vi "Olcme_Enstrumantasyon_Proje_170519035.vi"() -> ()   [LabVIEW 2021]
uses:
  <vilib>/Instr/_visa.llb/VISA Configure Serial Port (Instr).vi
panel:
  out "Z Ekseni İvme":dbl
  out "Y Ekseni İvme":dbl
  out "X Ekseni İvme":dbl
  out "Sıcaklık":dbl
  out "Okunan Değer":string
  in  "Seçilen COM":refnum<visa-resource-name>
  out "Z Ekseni İvme Grafiği":dbl(graph)
  out "Y Ekseni İvme Grafiği":dbl(graph)
  out "X Ekseni İvme Grafiği":dbl(graph)
  out "Sıcaklık Grafiği":dbl(graph)
  in  "stop":bool
  in  "baud rate (9600)":u32=9600
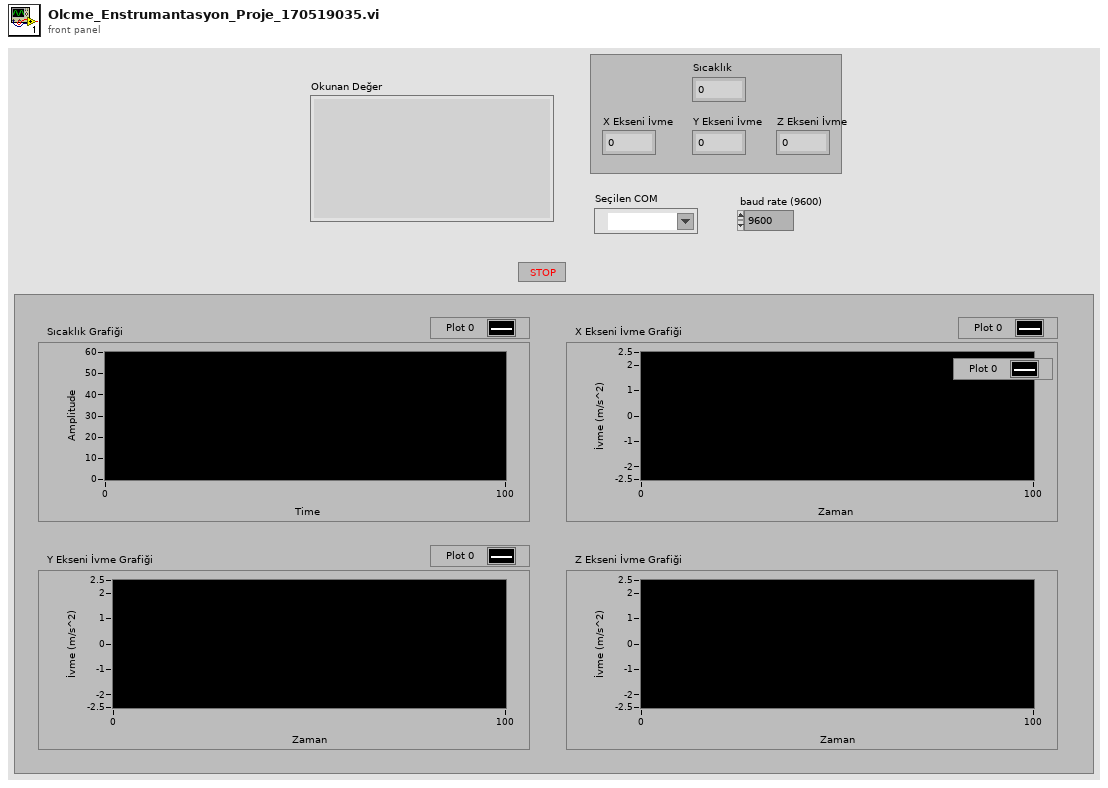
[diagram p1: front panel]
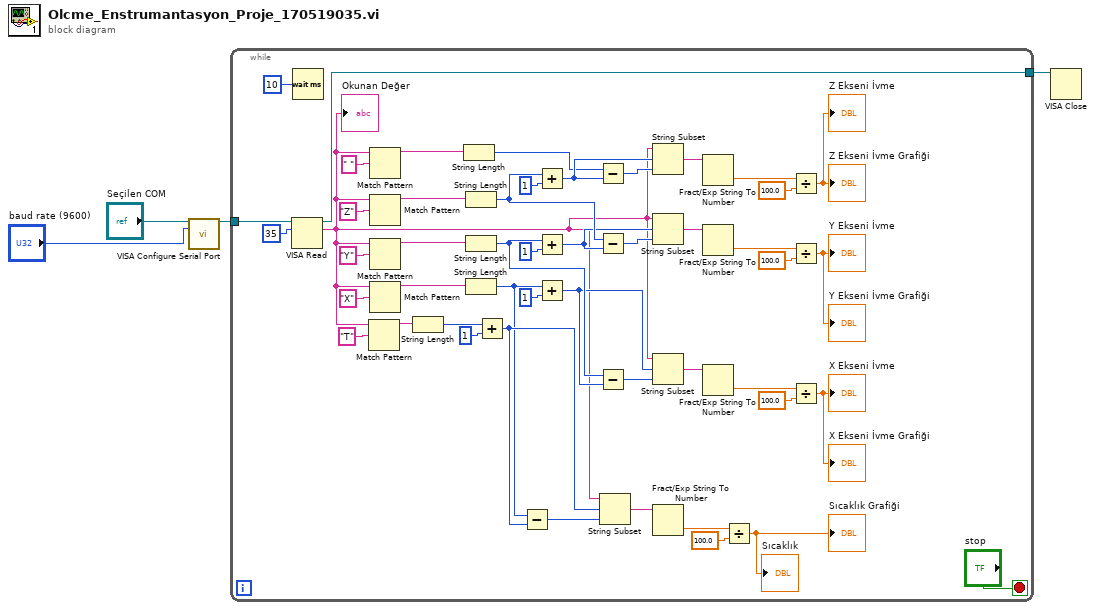
[diagram p0: block diagram]
diagram:
  n1 = call-poly "VISA Configure Serial Port"("VISA resource name"="Seçilen COM", "baud rate (9600)"="baud rate (9600)") -> ("VISA resource name out"=w3:refnum<visa-resource-name>)  [unwired: 12 in, 1 out]
  n2 = while {
    tunnel: w3 -> [w24]
    tunnel: [w22] -> w2
    stop <- "stop" stop-if-true
    n3 = VISA Read(VISA resource name=w24, byte count=u32 35) -> (VISA resource name out=w22:refnum<visa-resource-name>, read buffer=w9:string)  [unwired: 1 in, 2 out]
    "Okunan Değer" <- w9
    n4 = Wait (ms)(milliseconds to wait=u32 10) -> ()  [unwired: 1 out]
    n5 = Match Pattern(string=w9, regular expression="T") -> (before substring=w37:string)  [unwired: 1 in, 3 out]
    n6 = Match Pattern(string=w9, regular expression=" ") -> (before substring=w14:string)  [unwired: 1 in, 3 out]
    n7 = Match Pattern(string=w9, regular expression="Z") -> (before substring=w35:string)  [unwired: 1 in, 3 out]
    n8 = Match Pattern(string=w9, regular expression="Y") -> (before substring=w44:string)  [unwired: 1 in, 3 out]
    n9 = Match Pattern(string=w9, regular expression="X") -> (before substring=w47:string)  [unwired: 1 in, 3 out]
    n10 = String Length(string=w37) -> (length=w49:i32)
    n11 = String Length(string=w14) -> (length=w13:i32)
    n12 = String Length(string=w35) -> (length=w12:i32)
    n13 = String Length(string=w44) -> (length=w39:i32)
    n14 = String Length(string=w47) -> (length=w40:i32)
    n15 = Add(x=w49, y=1) -> (x+y=w46:i32)
    n16 = Subtract(x=w40, y=w46) -> (x-y=w34:i32)
    n17 = Add(x=w12, y=1) -> (x+y=w19:i32)
    n18 = Add(x=w39, y=1) -> (x+y=w11:i32)
    n19 = Add(x=w40, y=1) -> (x+y=w38:i32)
    n20 = Subtract(x=w13, y=w19) -> (x-y=w20:i32)
    n21 = Subtract(x=w12, y=w11) -> (x-y=w36:i32)
    n22 = Subtract(x=w39, y=w38) -> (x-y=w41:i32)
    n23 = String Subset(string=w9, offset (0)=w46, length (rest)=w34) -> (substring=w33:string)
    n24 = String Subset(string=w9, offset (0)=w19, length (rest)=w20) -> (substring=w18:string)
    n25 = String Subset(string=w9, offset (0)=w11, length (rest)=w36) -> (substring=w31:string)
    n26 = String Subset(string=w9, offset (0)=w38, length (rest)=w41) -> (substring=w32:string)
    n27 = Fract/Exp String To Number(string=w33) -> (number=w26:dbl)  [unwired: 3 in, 1 out]
    n28 = Fract/Exp String To Number(string=w18) -> (number=w17:dbl)  [unwired: 3 in, 1 out]
    n29 = Fract/Exp String To Number(string=w31) -> (number=w25:dbl)  [unwired: 3 in, 1 out]
    n30 = Fract/Exp String To Number(string=w32) -> (number=w27:dbl)  [unwired: 3 in, 1 out]
    n31 = Divide(x=w26, y=100.0) -> (x/y=→"Sıcaklık Grafiği" →"Sıcaklık":dbl)
    n32 = Divide(x=w17, y=100.0) -> (x/y=→"Z Ekseni İvme Grafiği" →"Z Ekseni İvme":dbl)
    n33 = Divide(x=w25, y=100.0) -> (x/y=→"Y Ekseni İvme Grafiği" →"Y Ekseni İvme":dbl)
    n34 = Divide(x=w27, y=100.0) -> (x/y=→"X Ekseni İvme Grafiği" →"X Ekseni İvme":dbl)
  }
  n35 = VISA Close(VISA resource name=w2) -> ()  [unwired: 1 in, 1 out]
